vi "Decode Packet.vi"(11 "IP Packet":u8[](array[numeric]) format="%02x") -> ()   [LabVIEW 2018]
panel:
  out "Destination Address":string
  out "Source Address":string
  out "Header Checksum":u16
  out "Protocol ID":u8
  out "TTL":u8
  out "Fragment Offset":u8
  out "Total Length (Bytes)":u16
  out "Flags":u8 format="%02x"
  out "ID":u16
  out "Type of Service":u8 format="%02x"
  out "IP Header Length (bytes)":u8
  out "IP Version":u8
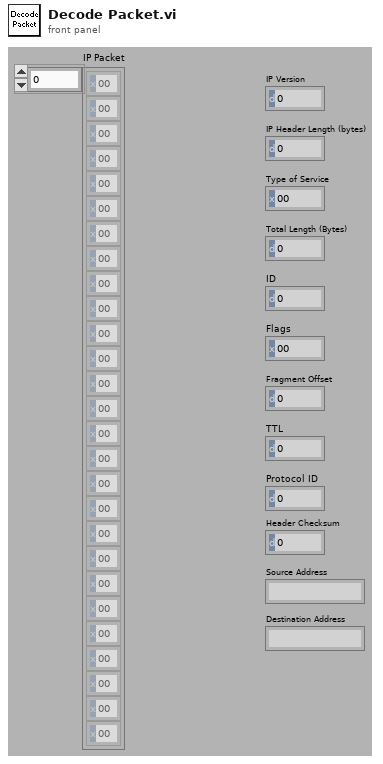
[diagram p1: front panel]
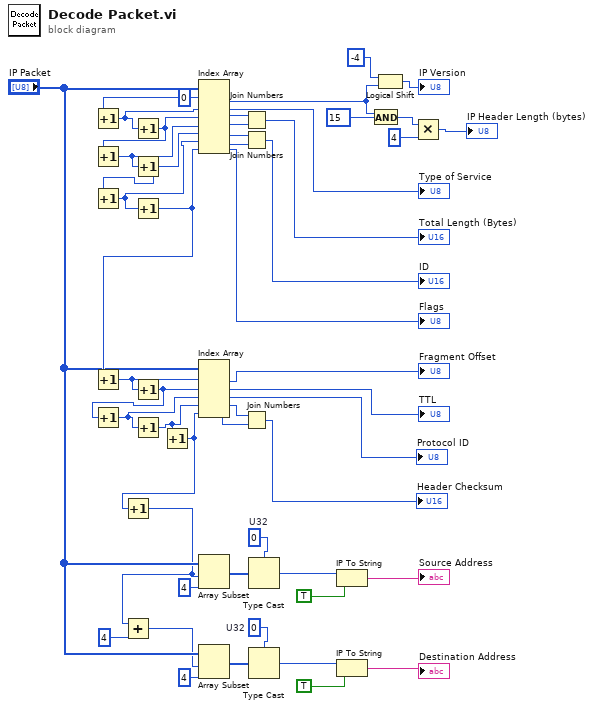
[diagram p0: block diagram]
diagram:
  w6 = u32 0  # U32
  w17 = u32 0  # U32
  w24 = 0 ("index")
  n1 = Increment(x=w24) -> (x+1=w23:i32)
  n2 = Increment(x=w23) -> (x+1=w22:i32)
  n3 = Increment(x=w22) -> (x+1=w21:i32)
  n4 = Increment(x=w21) -> (x+1=w20:i32)
  n5 = Increment(x=w20) -> (x+1=w19:i32)
  n6 = Increment(x=w19) -> (x+1=w18:i32)
  n7 = Increment(x=w18) -> (x+1=w32:i32)
  n8 = Increment(x=w32) -> (x+1=w31:i32)
  n9 = Increment(x=w31) -> (x+1=w30:i32)
  n10 = Increment(x=w30) -> (x+1=w28:i32)
  n11 = Increment(x=w28) -> (x+1=w15:i32)
  n12 = Increment(x=w15) -> (x+1=w2:i32)
  n13 = Add(x=w2, y=4) -> (x+y=w4:i32)
  n14 = Index Array(array="IP Packet", index #1=w24, index #2=w23, index #3=w22, index #4=w21, index #5=w20, index #6=w19, index #7=w18) -> (element #1=w47:u8, element #2=→"Type of Service":u8, element #3=w41:u8, element #4=w40:u8, element #5=w39:u8, element #6=w38:u8, element #7=→"Flags":u8)
  n15 = Index Array(array="IP Packet", index #1=w32, index #2=w31, index #3=w30, index #4=w28, index #5=w15) -> (element #1=→"Fragment Offset":u8, element #2=→"TTL":u8, element #3=→"Protocol ID":u8, element #4=w27:u8, element #5=w26:u8)
  n16 = Array Subset(array="IP Packet", index=w2, length=4) -> (w16:u8[])
  n17 = Array Subset(array="IP Packet", index=w4, length=4) -> (w7:u8[])
  n18 = Join Numbers(hi=w41, lo=w40) -> ((hi.lo)=→"Total Length (Bytes)":u16)
  n19 = Join Numbers(hi=w39, lo=w38) -> ((hi.lo)=→"ID":u16)
  n20 = Join Numbers(hi=w27, lo=w26) -> ((hi.lo)=→"Header Checksum":u16)
  n21 = Type Cast(type=w17, x=w16) -> (*(type *) &x=w13:u32)
  n22 = Type Cast(type=w6, x=w7) -> (*(type *) &x=w9:u32)
  n23 = IP To String(1:TRUE ("dot notation? (F)"), 2:w13) -> (0:→"Source Address":string)
  n24 = IP To String(1:TRUE ("dot notation? (F)"), 2:w9) -> (0:→"Destination Address":string)
  n25 = And(x=w47, y=u8 15) -> (x .and. y?=w45:u8)
  n26 = Logical Shift(y=-4, x=w47) -> (x << y=→"IP Version":u8)
  n27 = Multiply(x=w45, y=u8 4) -> (x*y=→"IP Header Length (bytes)":u8)
